vi "DBOpen-Error.vi"(8 "error in (no error)":errorcluster, 11 "ProcessState in":T1) -> (0 "error out":errorcluster, 3 "ProcessState out":T1)   [LabVIEW 2015, in "CopyUtility.lvlib"]
uses:
  CopyUtility.lvlib
  controls/ProcessState.ctl
  <vilib>/drjdpowell/SQLite Library/SQL Connection/Connection.lvclass
  DBToolkit/DBToolkit.lvlib
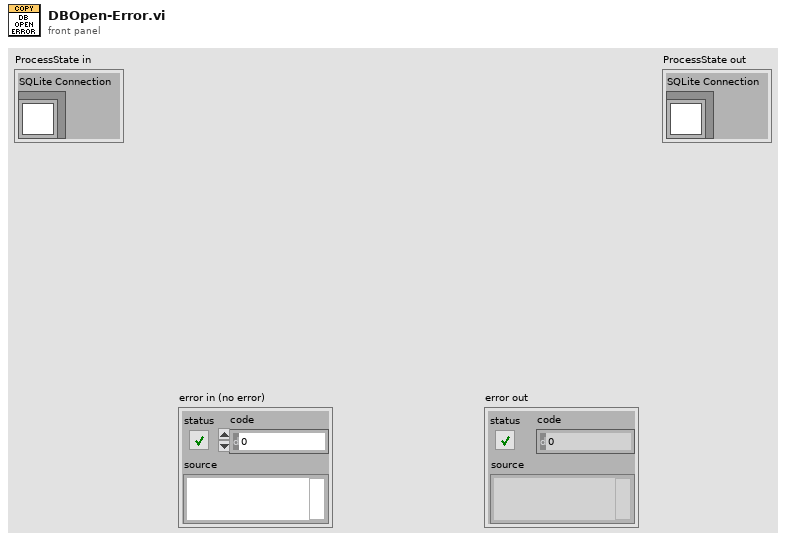
[diagram p1: front panel]
types:
  T1 = typedef "CopyUtility.lvlib/ProcessState.ctl" = cluster{"SQLite Connection":refnum<class "Connection.lvclass">}
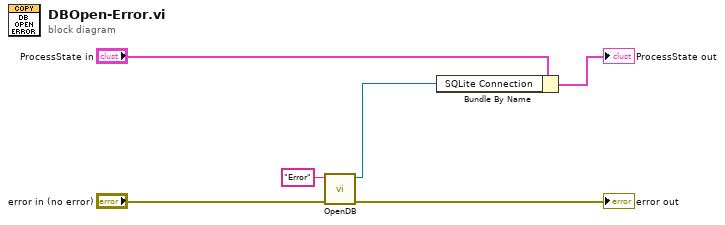
[diagram p0: block diagram]
diagram:
  n1 = call "OpenDB.vi"("error in (no error)"="error in (no error)", "DB File Name"="Error") -> ("error out"=→"error out":errorcluster, "SQLite Connection out"=w3:refnum<class "Connection.lvclass">)  [unwired: 8 in]
  n2 = Bundle By Name(cluster="ProcessState in", "SQLite Connection"=w3) -> (→"ProcessState out":T1)
